vi "graph_test.vi"() -> ()   [LabVIEW 2010]
panel:
  out "XY Graph":cluster{"Array 3":dbl[], "Array 2":dbl[]}[](graph)
  in  "Array 2":dbl[](array[numeric])
  in  "Array":dbl[](array[numeric])
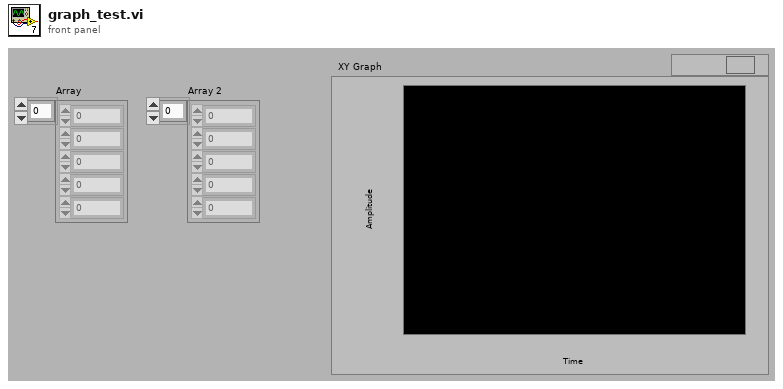
[diagram p1: front panel]
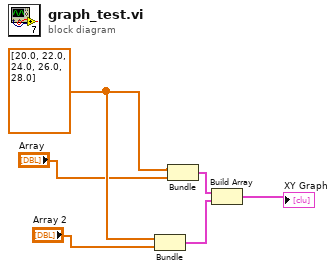
[diagram p0: block diagram]
diagram:
  w5 = dbl[] [20.0, 22.0, 24.0, 26.0, 28.0] ("Array 3")
  n1 = Bundle("Array 3"=w5, "Array 2"="Array 2") -> (w2:cluster{"Array 3":dbl[], "Array 2":dbl[]})  [unwired: 1 in]
  n2 = Bundle("Array 3"=w5, "Array"="Array") -> (w3:cluster{"Array 3":dbl[], "Array":dbl[]})  [unwired: 1 in]
  n3 = Build Array(w3, w2) -> (→"XY Graph":cluster{"Array 3":dbl[], "Array 2":dbl[]}[])
